vi "Delete FFT Plan 64f.vi"(8 "Error In":errorcluster, 11 "FFT Object":T1 {"Imag"."Dimension"."Width" min=1; "Imag"."Dimension"."Height" min=1; "Imag"."Dimension"."Depth" min=1; "Real"."Dimension"."Width" min=1; "Real"."Dimension"."Height" min=1; "Real"."Dimension"."Depth" min=1}) -> (0 "Error Out":errorcluster)   [LabVIEW 2012, in "OpenCLV x64.lvlib"]
doc: "Deletes the FFT plan and the associated memory objects."
uses:
  OpenCLV x64.lvlib
  FFT Control.ctl
  Controls/Device ID.ctl
  FFT Types.ctl
  FFT Dimension.ctl
  Controls/Memory Object.ctl
  Controls/Memory ID.ctl
  User Controls/Array Dimensions.ctl
  Controls/Memory Type.ctl
  FFT Direction.ctl
  Error Checking/Add Error Functional Global.vi
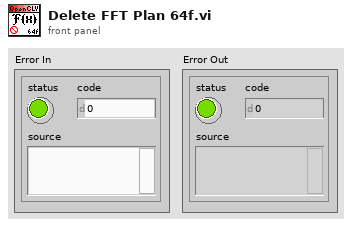
[diagram p1: front panel]
types:
  T1 = typedef "OpenCLV x64.lvlib/FFT Control.ctl" = cluster{"Device ID":T2, "FFT Types":T3, "FFT Dim":T4, "Real":T5, "Imag":T5, "FFT Plan":u64, "FFT Direction":T9}
  T2 = typedef "OpenCLV x64.lvlib/Device ID.ctl" = u64
  T3 = typedef "OpenCLV x64.lvlib/FFT Types.ctl" = enum16{"Real to Hermitian", "Hermitian to Real", "Complex to Complex"}
  T4 = typedef "OpenCLV x64.lvlib/FFT Dimension.ctl" = enum16{"1D FFT", "2D FFT", "3D FFT"}
  T5 = typedef "OpenCLV x64.lvlib/Memory Object.ctl" = cluster{"Device ID":T2, "Memeroy ID":T6, "Dimension":T7, "Memory Type":T8}
  T6 = typedef "OpenCLV x64.lvlib/Memory ID.ctl" = u64
  T7 = typedef "Array Dimensions.ctl" = cluster{"Depth":u64, "Height":u64, "Width":u64}
  T8 = typedef "OpenCLV x64.lvlib/Memory Type.ctl" = enum16{"32f", "u8", "i8", "u16", "i16", "u32", "i32", "64f"}
  T9 = typedef "OpenCLV x64.lvlib/FFT Direction.ctl" = enum16{"Forward", "Reverse"}
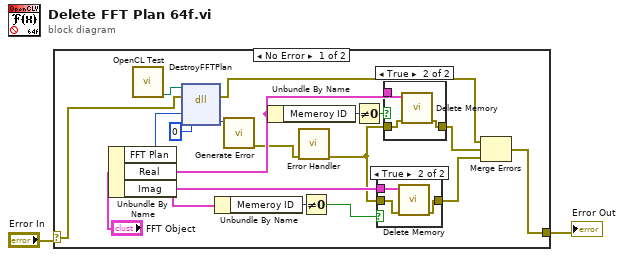
[diagram p0: block diagram]
diagram:
  n1 = case shown="No Error" "Error In" {
    selector: "Error In" -> [w3 w29]
    tunnel: [w15 w29] -> w1
    frame No Error {
      n2 = Unbundle By Name("FFT Object") -> ("FFT Plan"=w13:u64, "Real"=w7:T5, "Imag"=w11:T5)
      n3 = call "OpenCL Test.vi"() -> ("DLL To Use"=w6:path)  [unwired: 11 in]
      n4 = dll-call lib="C:/Users/bme-amcelroy-la/Desktop/OpenCLV/trunk/OpenCLV_x64_1.0/OpenCLV_x64.dll" fn="DestroyFFTPlan"(path in=w6, error in=w3, "FFT Plan"=w13, "Error"=0) -> (error out=w16:errorcluster, "Error"=w19:i32)  [unwired: 3 in, 1 out]
      n5 = Unbundle By Name(w11) -> ("Memeroy ID"=w12:T6)
      n6 = call "Generate Error.vi"("Error"=w19) -> ("error out"=w5:errorcluster)  [unwired: 10 in]
      n7 = Unbundle By Name(w7) -> ("Memeroy ID"=w9:T6)
      n8 = call-poly "Error Handler.vi"("Error In"=w5) -> ("Error Out"=w4:errorcluster)  [unwired: 10 in]
      n9 = Not Equal To 0?(x=w12) -> (x != 0?=w10:bool)
      n10 = Not Equal To 0?(x=w9) -> (x != 0?=w8:bool)
      n11 = case shown="True" w10 {
        tunnel: [w21 w24] -> w18
        tunnel: w11 -> [_ w23]
        tunnel: w4 -> [w21 w22]
        frame False {
        }
        frame True {
          n12 = call "Delete Memory.vi"("Error In"=w22, "Memory Object In"=w23) -> ("Error Out"=w24:errorcluster)  [unwired: 8 in, 1 out]
        }
      }
      n13 = case shown="True" w8 {
        tunnel: w4 -> [w25 w28]
        tunnel: [w25 w27] -> w17
        tunnel: w7 -> [_ w26]
        frame False {
        }
        frame True {
          n14 = call "Delete Memory.vi"("Error In"=w28, "Memory Object In"=w26) -> ("Error Out"=w27:errorcluster)  [unwired: 8 in, 1 out]
        }
      }
      n15 = Merge Errors(w16, w17, w18) -> (w15:errorcluster)
    }
    frame Error {
    }
  }
  "Error Out" <- w1
